vi "Polynomial follower 2.0.vi"() -> ()   [LabVIEW 2015]
uses:
  Polynomial First Derivitive.vi
  Polynomial.vi
  <vilib>/Rock Robotics/WPI/CAN/TalonSRX/WPI_CANTalonSRX_MotionProfileTrajectoryPt.ctl
  <vilib>/Rock Robotics/WPI/CAN/Jaguar/SubVIs/WPI_CANJaguar_ControlMode.ctl
  <vilib>/Rock Robotics/WPI/CAN/TalonSRX/WPI_CANTalonSRX_APIControlMode.ctl
  <vilib>/Rock Robotics/SystemInterfaces/DIO/FPGA_DIOPWMChannel.ctl
  <vilib>/Rock Robotics/WPI/PWM/WPI_PWMDeadband.ctl
  <vilib>/Rock Robotics/WPI/MotorControl/WPI_MotorControlType.ctl
  <vilib>/Rock Robotics/WPI/MotorControl/WPI_MotorControlDeviceRef.ctl
panel:
  in  "Talon Loop Time":dbl
  out "x*y":dbl
  in  "Robot Width":dbl=21.5
  in  "Resolution":dbl=0.001
  in  "Initial Acceleration":T1
  in  "Initial Velocities (1 to (-1))":T2
  in  "Max Velocity in/s":dbl
  in  "Max acceleration in/s^2":dbl
  in  "Max Jerk in/s^3":dbl
  in  "CAN Talon SRX Ref Left":T3={"DeviceStatus"={"status"=FALSE, "code"=0, "source"=""}, "Type"=enum."PWM", "PWM"={"PWM Channel"=enum."PWM 1", "DeadBand"={"Name"="", "maxPositivePwm"=0, "minPositivePwm"=0, "centerPwm"=0, "maxNegativePwm"=0, "minNegativePwm"=0, "angularRange"=0}}, "CAN"={"Device Number"=0, "Control Mode"=enum."Percent VBus", "Semaphore"=refnum, "Max Vout"=12.0, "TalonSRX Control Mode"=enum."Percent VBus"}, "Invert"=FALSE}
  in  "CAN Talon SRX Ref Right":T3={"DeviceStatus"={"status"=FALSE, "code"=0, "source"=""}, "Type"=enum."PWM", "PWM"={"PWM Channel"=enum."PWM 1", "DeadBand"={"Name"="", "maxPositivePwm"=0, "minPositivePwm"=0, "centerPwm"=0, "maxNegativePwm"=0, "minNegativePwm"=0, "angularRange"=0}}, "CAN"={"Device Number"=0, "Control Mode"=enum."Percent VBus", "Semaphore"=refnum, "Max Vout"=12.0, "TalonSRX Control Mode"=enum."Percent VBus"}, "Invert"=FALSE}
  in  "Right bound":dbl
  in  "Polynomial":dbl[](array[numeric])
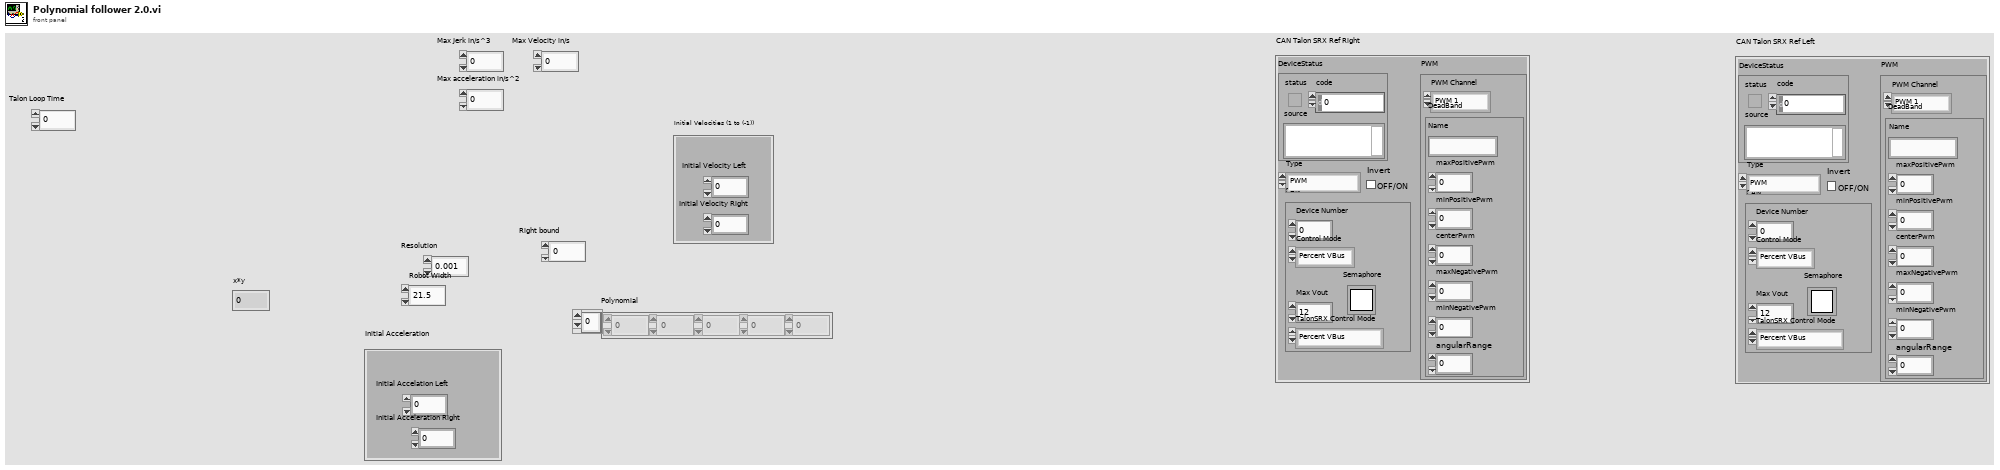
[diagram p1: front panel]
types:
  T1 = cluster{"Initial Accelation Left":dbl, "Initial Acceleration Right":dbl}
  T2 = cluster{"Initial Velocity Left":dbl, "Initial Velocity Right":dbl}
  T3 = typedef "WPI_MotorControlDeviceRef.ctl" = cluster{"DeviceStatus":errorcluster, "Type":T4, "PWM":cluster{"PWM Channel":T5, "DeadBand":T6}, "CAN":cluster{"Device Number":u8, "Control Mode":T7, "Semaphore":T8, "Max Vout":dbl, "TalonSRX Control Mode":T9}, "Invert":bool}
  T4 = typedef "WPI_MotorControlType.ctl" = enum16{"PWM", "CAN", "CANTalonSRX"}
  T5 = typedef "FPGA_DIOPWMChannel.ctl" = enum8{"PWM 0", "PWM 1", "PWM 2", "PWM 3", "PWM 4", "PWM 5", "PWM 6", "PWM 7", "PWM 8", "PWM 9", "PWM MXP 0", "PWM MXP 1", "PWM MXP 2", "PWM MXP 3", "PWM MXP 4", "PWM MXP 5", "PWM MXP 6", "PWM MXP 7", "PWM MXP 8", "PWM MXP 9", "Invalid"}
  T6 = typedef "WPI_PWMDeadband.ctl" = cluster{"Name":string, "maxPositivePwm":i32, "minPositivePwm":i32, "centerPwm":i32, "maxNegativePwm":i32, "minNegativePwm":i32, "angularRange":u16}
  T7 = typedef "WPI_CANJaguar_ControlMode.ctl" = enum8{"Percent VBus", "Current", "Speed", "Position", "Voltage"}
  T8 = typedef "Semaphore RefNum" = refnum<k1>
  T9 = typedef "WPI_CANTalonSRX_APIControlMode.ctl" = enum8{"Percent VBus", "Speed", "Position", "Slave", "Unchanged / Invalid", "Voltage Compensation", "Current", "Motion Profile"}
  T10 = typedef "WPI_CANTalonSRX_MotionProfileTrajectoryPt.ctl" = cluster{"Duration Ms":u8, "Velocity":dbl, "Position":dbl, "Profile Slot Select":u8, "Is Last":bool, "Velocity Only":bool, "Zero Position":bool, "Compress Code":u8, "Same Velocity":i32, "Delta Position":i32, "Count":u8}
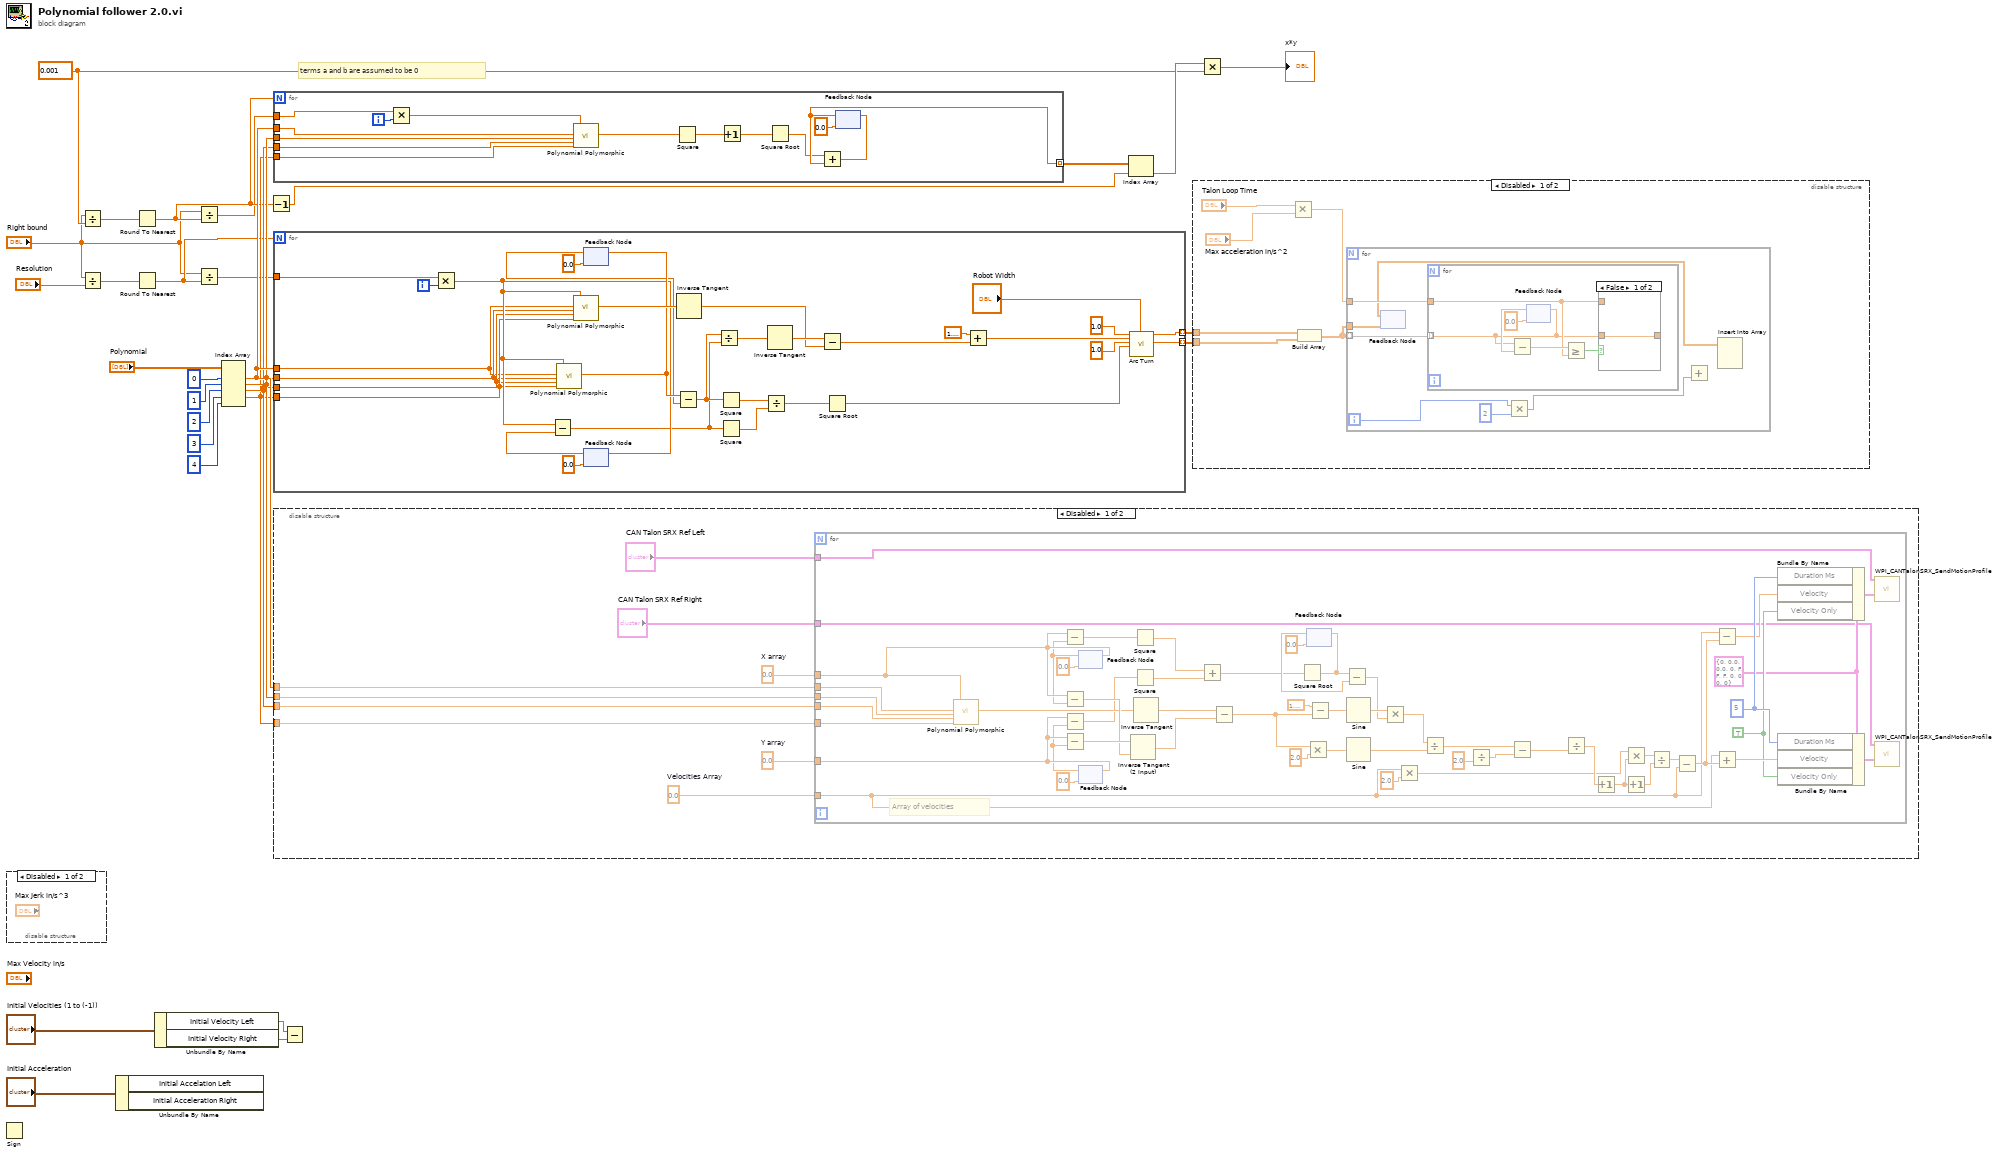
[diagram p0: block diagram]
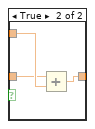
[diagram p2: hidden frame]
diagram:
  w19 = 0.001
  # "terms a and b are assumed to be 0"
  n1 = Sign() -> ()  [unwired: 1 in, 1 out]
  n2 = disable-structure shown="Disabled" {
    frame Disabled {
    }
    frame Enabled {
    }
  }
  n3 = Divide(x="Right bound", y=w19) -> (x/y=w24:dbl)
  n4 = Divide(x="Right bound", y="Resolution") -> (x/y=w12:dbl)
  n5 = Unbundle By Name("Initial Acceleration") -> ()  [unwired: 2 out]
  n6 = Round To Nearest(number=w24) -> (nearest integer value=w8:dbl)
  n7 = Round To Nearest(number=w12) -> (nearest integer value=w10:dbl)
  n8 = Unbundle By Name("Initial Velocities (1 to (-1))") -> ("Initial Velocity Left"=w4:dbl, "Initial Velocity Right"=w3:dbl)
  n9 = Divide(x="Right bound", y=w8) -> (x/y=w6:dbl)
  n10 = Divide(x="Right bound", y=w10) -> (x/y=w9:dbl)
  n11 = Index Array(array="Polynomial", index #1=0 ("index"), index #2=1 ("index"), index #3=2 ("index"), index #4=3 ("index"), index #5=4) -> (element #1=w16:dbl, element #2=w15:dbl, element #3=w14:dbl, element #4=w13:dbl)  [unwired: 1 out]
  n12 = Decrement(x=w8) -> (x-1=w21:dbl)
  n13 = for {
    N: w8 -> [_]
    tunnel: w16 -> [w30]
    tunnel: w15 -> [w31]
    tunnel: w14 -> [w32]
    tunnel: w13 -> [w33]
    tunnel: w6 -> [w42]
    tunnel: [w38] -> w22 mode=indexing
    i -> [w43]
    n14 = Multiply(x=w42, y=w43) -> (x*y=w41:dbl)
    n15 = call-poly "Polynomial Polymorphic.vi"("CX^2"=w30, "DX^3"=w31, "EX^4"=w32, "FX^5"=w33, "X"=w41) -> ("Y"=w37:dbl)  [unwired: 14 in]
    n16 = Square(x=w37) -> (x^2=w36:dbl)
    n17 = Increment(x=w36) -> (x+1=w35:dbl)
    n18 = Square Root(x=w35) -> (sqrt(x)=w34:dbl)
    n19 = feedback #1(0.0) -> (w38:dbl)
    n20 = Add(x=w34, y=w38) -> (x+y=w40:dbl)
    n21 = feedback-in #1(w40) -> ()
  }
  n22 = for {
    N: w10 -> [_]
    tunnel: w16 -> [w46]
    tunnel: w15 -> [w47]
    tunnel: w14 -> [w48]
    tunnel: w13 -> [w49]
    tunnel: w9 -> [w71]
    tunnel: [w45] -> w2 mode=indexing
    tunnel: [w44] -> w1 mode=indexing
    i -> [w72]
    n23 = Multiply(x=w71, y=w72) -> (x*y=w65:dbl)
    n24 = call-poly "Polynomial Polymorphic.vi"("CX^2"=w46, "DX^3"=w47, "EX^4"=w48, "FX^5"=w49, "X"=w65) -> ("Y"=w70:dbl)  [unwired: 14 in]
    n25 = call-poly "Polynomial Polymorphic.vi"("CX^2"=w46, "DX^3"=w47, "EX^4"=w48, "FX^5"=w49, "X"=w65) -> ("Y"=w73:dbl)  [unwired: 14 in]
    n26 = feedback-in #2(w70) -> ()
    n27 = feedback #2(0.0 ("Y")) -> (w69:dbl)
    n28 = feedback #3(0.0 ("Y")) -> (w67:dbl)
    n29 = Subtract(x=w65, y=w67) -> (x-y=w62:dbl)
    n30 = feedback-in #3(w65) -> ()
    n31 = Subtract(x=w70, y=w69) -> (x-y=w63:dbl)
    n32 = Inverse Tangent(1:w73) -> (0:w54:dbl)
    n33 = Divide(x=w63, y=w62) -> (x/y=w64:dbl)
    n34 = Square(x=w63) -> (x^2=w61:dbl)
    n35 = Square(x=w62) -> (x^2=w60:dbl)
    n36 = Divide(x=w61, y=w60) -> (x/y=w59:dbl)
    n37 = Inverse Tangent(1:w64) -> (0:w55:dbl)
    n38 = Subtract(x=w55, y=w54) -> (x-y=w53:dbl)
    n39 = Square Root(x=w59) -> (sqrt(x)=w58:dbl)
    n40 = Add(x=1.5707963267948966, y=w53) -> (x+y=w57:dbl)
    n41 = call "Arc Turn.vi"("Speed Setpoint (0-1)"=1.0, "Angle Radians (0 = Right)"=w57, "Max Speed (TPS)"=1.0, "Distance"=w58, "Robot Width"="Robot Width") -> ("Left Speed"=w45:dbl, "Right Speed"=w44:dbl)  [unwired: 13 in]
  }
  n42 = disable-structure shown="Disabled" {
    disable-tunnel: w16 -> [w77 _]
    disable-tunnel: w15 -> [w76 _]
    disable-tunnel: w14 -> [w75 _]
    disable-tunnel: w13 -> [w74 _]
    frame Disabled {
      w80 = 0.0  # Y array
      w81 = 0.0  # Velocities Array
      w82 = 0.0  # X array
      n43 = for {
        tunnel: w81 -> [w97]
        tunnel: w82 -> [w103]
        tunnel: w77 -> [w83]
        tunnel: w76 -> [w84]
        tunnel: w75 -> [w85]
        tunnel: w74 -> [w86]
        tunnel: w80 -> [w107]
        tunnel: "CAN Talon SRX Ref Left" -> [w89]
        tunnel: "CAN Talon SRX Ref Right" -> [w88]
        w92 = T10 {"Duration Ms"=0, "Velocity"=0.0, "Position"=0.0, "Profile Slot Select"=0, "Is Last"=FALSE, "Velocity Only"=FALSE, "Zero Position"=FALSE, "Compress Code"=0, "Same Velocity"=0, "Delta Position"=0, "Count"=0} ("New Point")
        w96 = u8 5 ("Duration Ms")
        w93 = TRUE
        # "Array of velocities"
        n44 = call-poly "Polynomial Polymorphic.vi"("CX^2"=w83, "DX^3"=w84, "EX^4"=w85, "FX^5"=w86, "X"=w103) -> ("Y"=w110:dbl)  [unwired: 14 in]
        n45 = feedback #4(0.0 ("Cumulative Distances Array")) -> (w102:dbl)
        n46 = Subtract(x=w103, y=w102) -> (x-y=w104:dbl)
        n47 = Subtract(x=w103, y=w102) -> (x-y=w111:dbl)
        n48 = feedback-in #4(w103) -> ()
        n49 = feedback #5(0.0 ("Cumulative Distances Array")) -> (w106:dbl)
        n50 = Subtract(x=w107, y=w106) -> (x-y=w105:dbl)
        n51 = Subtract(x=w107, y=w106) -> (x-y=w112:dbl)
        n52 = feedback-in #5(w107) -> ()
        n53 = Inverse Tangent (2 Input)(1:w111, 2:w112) -> (0:w108:dbl)
        n54 = Square(x=w104) -> (x^2=w101:dbl)
        n55 = Square(x=w105) -> (x^2=w100:dbl)
        n56 = Inverse Tangent(1:w110) -> (0:w109:dbl)
        n57 = Add(x=w101, y=w100) -> (x+y=w99:dbl)
        n58 = Subtract(x=w109, y=w108) -> (x-y=w87:dbl)
        n59 = Square Root(x=w99) -> (sqrt(x)=w98:dbl)
        n60 = Multiply(x=w87, y=2.0) -> (x*y=w131:dbl)
        n61 = feedback-in #6(w98) -> ()
        n62 = feedback #6(0.0 ("Cumulative Distances Array")) -> (w116:dbl)
        n63 = Subtract(x=1.5707963267948966, y=w87) -> (x-y=w135:dbl)
        n64 = Subtract(x=w98, y=w116) -> (x-y=w115:dbl)
        n65 = Sine(x=w135) -> (sin(x)=w134:dbl)
        n66 = Sine(x=w131) -> (sin(x)=w130:dbl)
        n67 = Multiply(x=w134, y=w115) -> (x*y=w133:dbl)
        n68 = Multiply(x=w97, y=2.0) -> (x*y=w124:dbl)
        n69 = Divide(x=w133, y=w130) -> (x/y=w129:dbl)
        n70 = Divide(y=2.0) -> (x/y=w118:dbl)  [unwired: 1 in]
        n71 = Subtract(x=w129, y=w118) -> (x-y=w128:dbl)
        n72 = Divide(y=w128) -> (x/y=w127:dbl)  [unwired: 1 in]
        n73 = Increment(x=w127) -> (x+1=w122:dbl)
        n74 = Multiply(x=w124, y=w122) -> (x*y=w123:dbl)
        n75 = Increment(x=w122) -> (x+1=w121:dbl)
        n76 = Divide(x=w123, y=w121) -> (x/y=w120:dbl)
        n77 = Subtract(x=w120, y=w97) -> (x-y=w119:dbl)
        n78 = Subtract(x=w97, y=w119) -> (x-y=w95:dbl)
        n79 = Add(x=w97, y=w119) -> (x+y=w94:dbl)
        n80 = Bundle By Name(cluster=w92, "Duration Ms"=w96, "Velocity"=w95, "Velocity Only"=w93) -> (w91:T10)
        n81 = Bundle By Name(cluster=w92, "Duration Ms"=w96, "Velocity"=w94, "Velocity Only"=w93) -> (w90:T10)
        n82 = call <vilib>:"WPI_CANTalonSRX_SendMotionProfile.vi"("CAN Talon SRX Ref"=w89, "New Point"=w91) -> ()  [unwired: 10 in, 4 out]
        n83 = call <vilib>:"WPI_CANTalonSRX_SendMotionProfile.vi"("CAN Talon SRX Ref"=w88, "New Point"=w90) -> ()  [unwired: 10 in, 4 out]
      }
    }
    frame Enabled {
    }
  }
  n84 = Subtract(x=w4, y=w3) -> ()  [unwired: 1 out]
  n85 = Index Array(array=w22, index=w21) -> (element=w20:dbl)
  n86 = disable-structure shown="Disabled" {
    disable-tunnel: w2 -> [w142 _]
    disable-tunnel: w1 -> [w141 _]
    frame Disabled {
      n87 = Multiply(x="Talon Loop Time", y="Max acceleration in/s^2") -> (x*y=w138:dbl)
      n88 = Build Array(w142, w141) -> (w137:dbl[][])
      n89 = for {
        tunnel: w137 -> [w147] mode=indexing
        tunnel: w138 -> [w148]
        tunnel: w137 -> [w149]
        i -> [w144]
        n90 = feedback #7(w149) -> (w146:dbl[][])
        n91 = feedback-in #7() -> ()  [unwired: 1 out]
        n92 = for {
          tunnel: w148 -> [w152]
          tunnel: w147 -> [w150] mode=indexing
          n93 = feedback #8(0.0 ("Right Speed")) -> (w155:dbl)
          n94 = Subtract(x=w150, y=w155) -> (x-y=w153:dbl)
          n95 = feedback-in #8(w150) -> ()
          n96 = Greater Or Equal?(x=w153, y=w152) -> (x >= y?=w154:bool)
          n97 = case shown="False" w154 {
            tunnel: w152 -> [_ w159]
            tunnel: w150 -> [w156 w158]
            tunnel: [w156 w157] -> _
            frame False {
            }
            frame True {
              n98 = Add(x=w158, y=w159) -> (x+y=w157:dbl)
            }
          }
        }
        n99 = Multiply(x=w144, y=2) -> (x*y=w143:i32)
        n100 = Add(y=w143) -> ()  [unwired: 1 in, 1 out]
        n101 = Insert Into Array(array=w146) -> ()  [unwired: 3 in, 1 out]
      }
    }
    frame Enabled {
    }
  }
  n102 = Multiply(x=w20, y=w19) -> (x*y=→"x*y":dbl)
